vi "hamamatsu_dcam_update_camera_settings.vi"(6 "error in (no error)":errorcluster, 9 "Handle in":u32) -> (0 "error out":errorcluster, 3 "Handle out":u32)   [LabVIEW 2015]
panel:
  out "Display":T1(plugin-control)
  out "Software FPS":dbl
  out "Camera FPS":dbl
  out "SMD":dbl
  in  "Scan Mode":dbl min=1.0 max=2.0 step=1.0
  in  "Exposure":dbl min=0.0010036691729323308 max=10.000004210526315 step=1e-08
  out "EXP":dbl
  out "SVW":i32
  out "SHW":i32
  out "SVO":i32
  out "SHO":i32
  in  "V Width":i32 min=4 max=1124 step=4
  in  "V Offset":i32 min=0 max=1848 step=4
  in  "H Width":i32 min=4 max=2048 step=4
  in  "H Offset":i32 min=0 max=0 step=4
  in  "Binning":u16(ring)=1 items=["1x1"=1, "2x2"=2, "4x4"=4]
  out "Elapsed Time":u32
  out "Total Frames":i32
  in  "Display":bool=TRUE
  in  "continue":bool
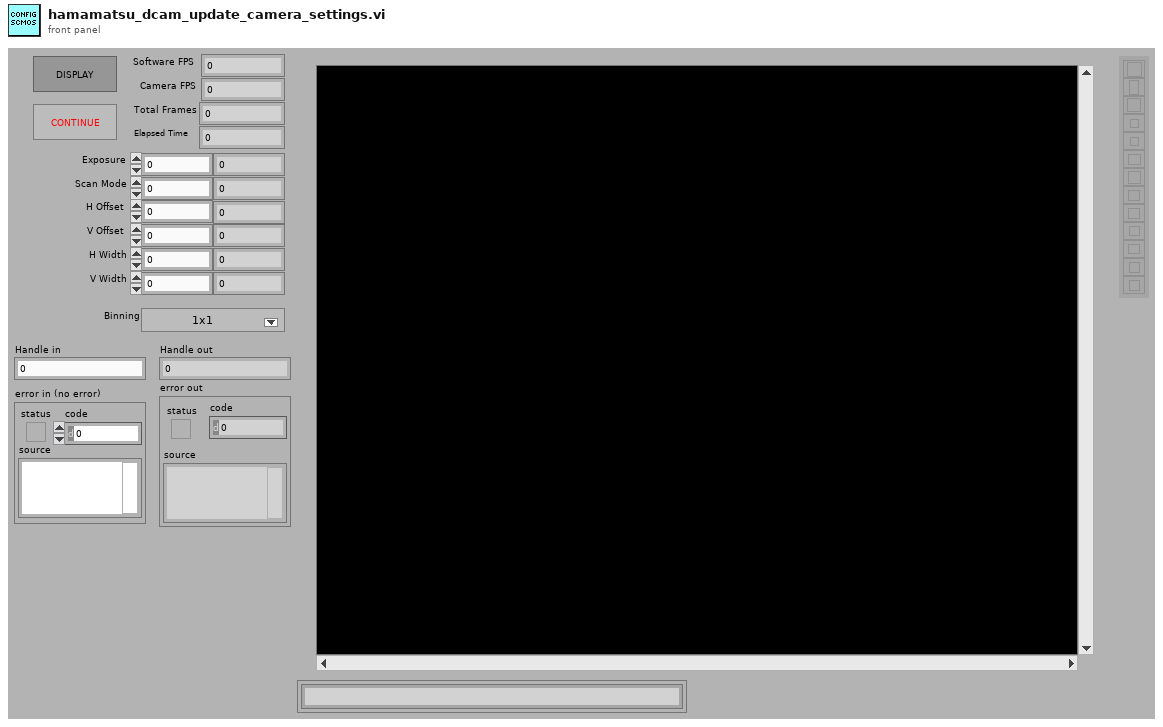
[diagram p1: front panel]
types:
  T1 = typedef "IMAQ Image.ctl" = refnum<image>
  T2 = typedef "Image Type" = u32
  T3 = cluster{"Value":i32, "Minimum":i32, "Maximum":i32, "Increment":i32}
  T4 = cluster{"height":u32, "width":u32, "datatype":u32}
  T5 = cluster{"H Offset":i32, "V Offset":i32, "H Width":i32, "V Width":i32}
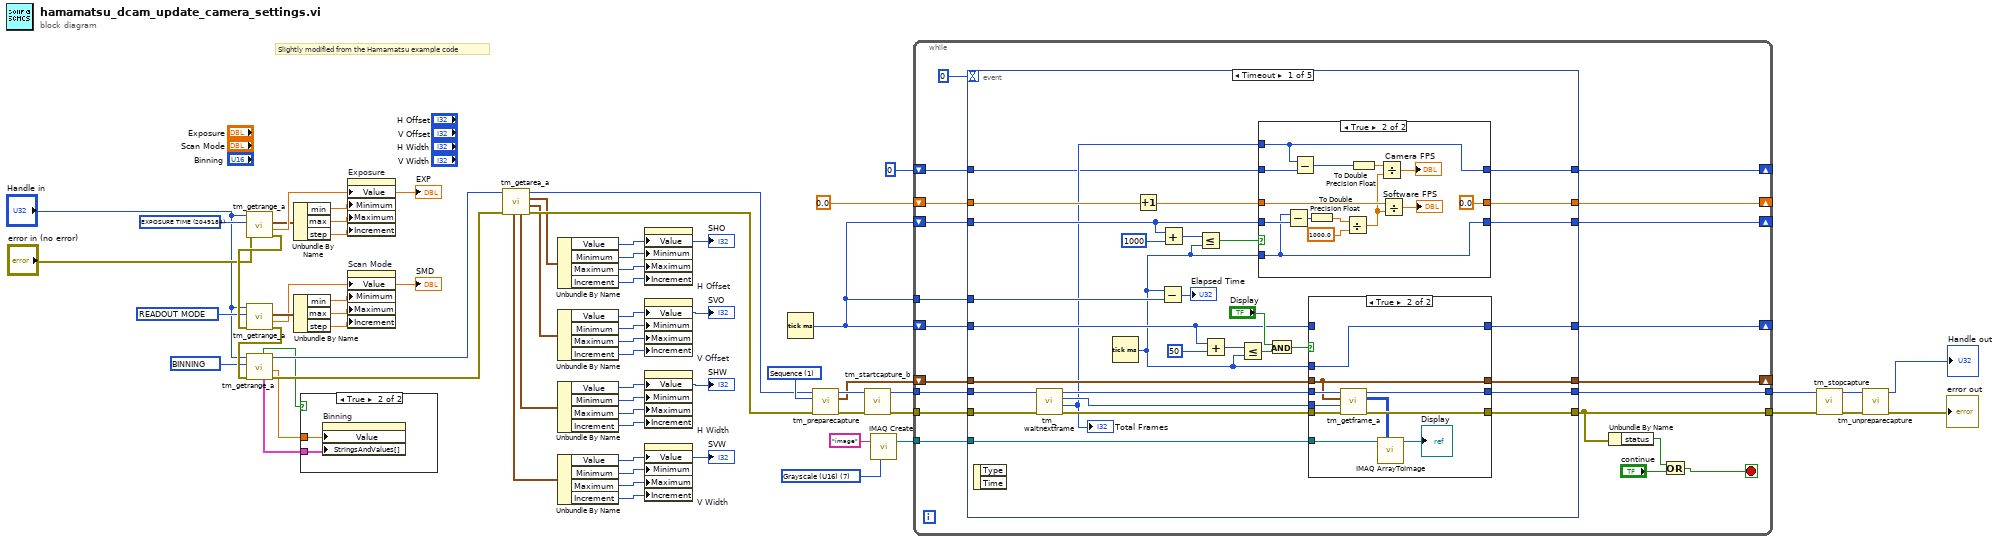
[diagram p0: block diagram]
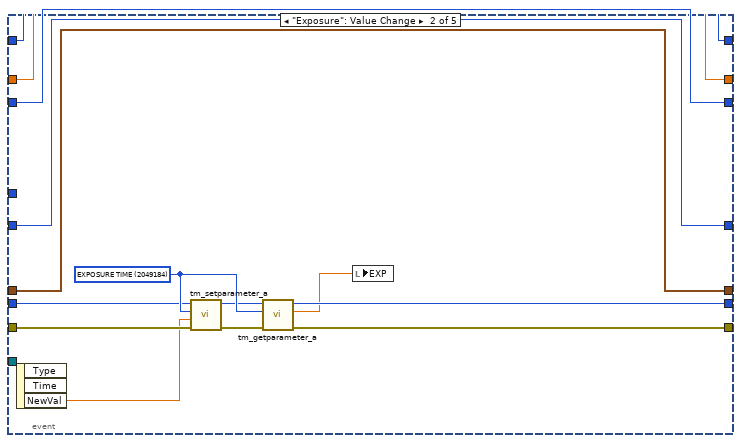
[diagram p5: hidden frame]
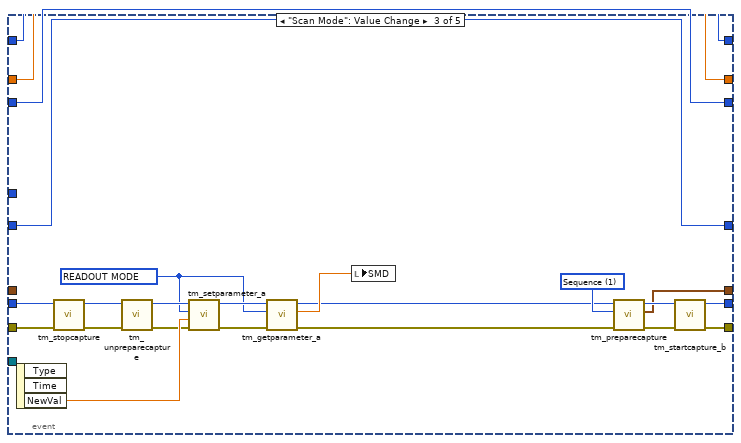
[diagram p6: hidden frame]
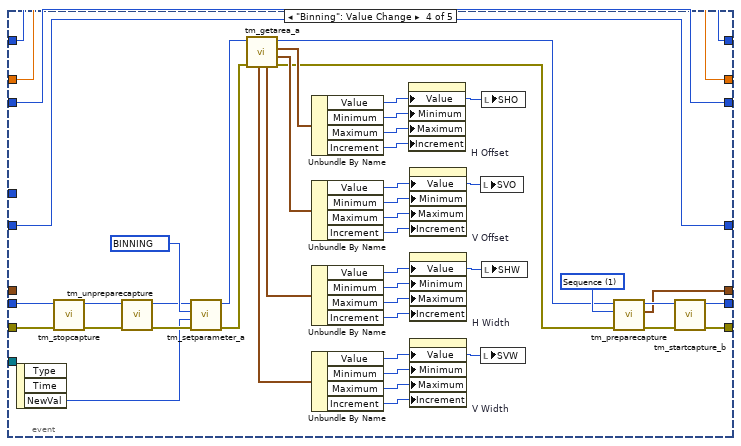
[diagram p7: hidden frame]
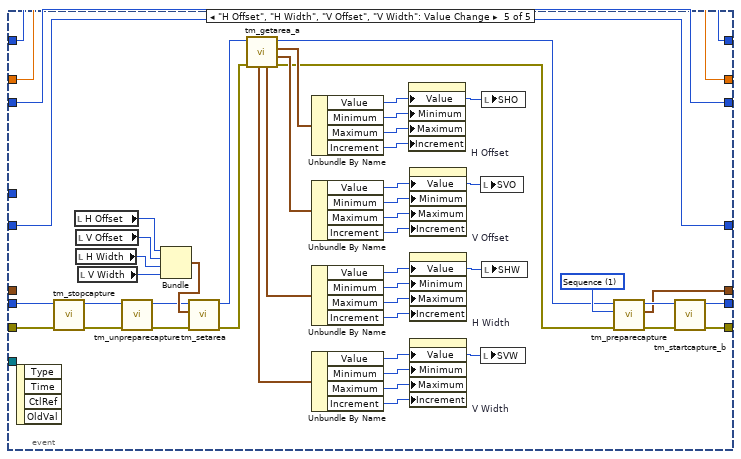
[diagram p8: hidden frame]
diagram:
  w8 = T2 7 items=["Grayscale (U8)", "Grayscale (I16)", "Grayscale (SGL)", "Complex (CSG)", "RGB (U32)", "HSL (U32)", "RGB (U64)", "Grayscale (U16)"] ("Image Type")
  w10 = u32 2049184 items=["BINNING"=4215968, "BITS PER CHANNEL"=4342976, "ACTIVE VIEW INDEX"=4343136, "CCD MODE"=4212384, "SENSOR MODE"=4212128, "READOUT MODE"=4211872, "EXPOSURE TIME"=2049184, "CONTRAST GAIN"=3163312, "CONTRAST OFFSET"=3163328, "LIGHT MODE"=2114720, "SENSITIVITY"=2114992, "WHITE BALANCE"=3163568, "PHOTON IMAGING MODE"=2115200, "HIGH DYNAMIC RANGE MODE"=3163360, "TRIGGER SOURCE"=1066144, "TRIGGER ACTIVE"=1066160, "TRIGGER MODE"=1066400, "TRIGGER POLARITY"=1066416, "TRIGGER GLOBAL EXPOSURE"=2049680, "FIRST TRIGGER BEHAVIOR"=2049696, "TRIGGER TIMES"=1066448, "OUTPUT TRIGGER POLARITY"=1852592, "OUTPUT TRIGGER DELAY"=1852624, "OUTPUT TRIGGER PERIOD"=1852640, "TEMPERATURE"=2115232, "TEMPERATURE TARGET"=2115264, "SENSOR COOLER FAN"=2115296, "MECHANICAL SHUTTER"=2115488, "BACK FOCUS POSITION"=8422304, "FRAMEBUNDLE MODE"=4346784, "FRAMEBUNDLE NUMBER"=4346800, "LINEBUNDLE HEIGHT"=4212192, "TRIGGER CONNECTOR"=1066432, "IMAGE PIXEL TYPE"=4343296, "OUTPUT TRIGGER KIND"=1852656, "READOUT DIRECTION"=4211904, "CHANNEL SYNC"=1852352] ("Parameter")
  w11 = u32 4211872 items=["BINNING"=4215968, "BITS PER CHANNEL"=4342976, "ACTIVE VIEW INDEX"=4343136, "CCD MODE"=4212384, "SENSOR MODE"=4212128, "READOUT MODE"=4211872, "EXPOSURE TIME"=2049184, "CONTRAST GAIN"=3163312, "CONTRAST OFFSET"=3163328, "LIGHT MODE"=2114720, "SENSITIVITY"=2114992, "WHITE BALANCE"=3163568, "PHOTON IMAGING MODE"=2115200, "HIGH DYNAMIC RANGE MODE"=3163360, "TRIGGER SOURCE"=1066144, "TRIGGER ACTIVE"=1066160, "TRIGGER MODE"=1066400, "TRIGGER POLARITY"=1066416, "TRIGGER GLOBAL EXPOSURE"=2049680, "FIRST TRIGGER BEHAVIOR"=2049696, "TRIGGER TIMES"=1066448, "OUTPUT TRIGGER POLARITY"=1852592, "OUTPUT TRIGGER DELAY"=1852624, "OUTPUT TRIGGER PERIOD"=1852640, "TEMPERATURE"=2115232, "TEMPERATURE TARGET"=2115264, "SENSOR COOLER FAN"=2115296, "MECHANICAL SHUTTER"=2115488, "BACK FOCUS POSITION"=8422304, "FRAMEBUNDLE MODE"=4346784, "FRAMEBUNDLE NUMBER"=4346800, "LINEBUNDLE HEIGHT"=4212192, "TRIGGER CONNECTOR"=1066432, "IMAGE PIXEL TYPE"=4343296, "OUTPUT TRIGGER KIND"=1852656, "READOUT DIRECTION"=4211904, "CHANNEL SYNC"=1852352] ("Parameter")
  w12 = u32 4215968 items=["BINNING"=4215968, "BITS PER CHANNEL"=4342976, "ACTIVE VIEW INDEX"=4343136, "CCD MODE"=4212384, "SENSOR MODE"=4212128, "READOUT MODE"=4211872, "EXPOSURE TIME"=2049184, "CONTRAST GAIN"=3163312, "CONTRAST OFFSET"=3163328, "LIGHT MODE"=2114720, "SENSITIVITY"=2114992, "WHITE BALANCE"=3163568, "PHOTON IMAGING MODE"=2115200, "HIGH DYNAMIC RANGE MODE"=3163360, "TRIGGER SOURCE"=1066144, "TRIGGER ACTIVE"=1066160, "TRIGGER MODE"=1066400, "TRIGGER POLARITY"=1066416, "TRIGGER GLOBAL EXPOSURE"=2049680, "FIRST TRIGGER BEHAVIOR"=2049696, "TRIGGER TIMES"=1066448, "OUTPUT TRIGGER POLARITY"=1852592, "OUTPUT TRIGGER DELAY"=1852624, "OUTPUT TRIGGER PERIOD"=1852640, "TEMPERATURE"=2115232, "TEMPERATURE TARGET"=2115264, "SENSOR COOLER FAN"=2115296, "MECHANICAL SHUTTER"=2115488, "BACK FOCUS POSITION"=8422304, "FRAMEBUNDLE MODE"=4346784, "FRAMEBUNDLE NUMBER"=4346800, "LINEBUNDLE HEIGHT"=4212192, "TRIGGER CONNECTOR"=1066432, "IMAGE PIXEL TYPE"=4343296, "OUTPUT TRIGGER KIND"=1852656, "READOUT DIRECTION"=4211904, "CHANNEL SYNC"=1852352] ("Parameter")
  w61 = 1 items=["Snap", "Sequence"] ("Capture mode")
  # "Slightly modified from the Hamamatsu example code"
  n1 = call <userlib>:"tm_getrange_a.vi"("error in (no error)"="error in (no error)", "Parameter"=w10, "Handle in"="Handle in") -> ("error out"=w21:errorcluster, "default"=w23:dbl, "Range"=w22:cluster{"min":dbl, "max":dbl, "step":dbl})  [unwired: 2 in, 4 out]
  "EXP" <- w23
  n2 = call <userlib>:"tm_getrange_a.vi"("error in (no error)"=w21, "Parameter"=w11, "Handle in"="Handle in") -> ("error out"=w18:errorcluster, "default"=w19:dbl, "Range"=w20:cluster{"min":dbl, "max":dbl, "step":dbl})  [unwired: 2 in, 4 out]
  "SMD" <- w19
  n3 = call <userlib>:"tm_getrange_a.vi"("error in (no error)"=w18, "Parameter"=w12, "Handle in"="Handle in") -> ("error out"=w17:errorcluster, "default"=w14:dbl, "Handle out"=w16:u32, "Value Names"=w13:cluster{"Name":string, "Value":dbl}[], "Writable"=w15:bool)  [unwired: 2 in, 2 out]
  n4 = Unbundle By Name(w22) -> ("min"=w54:dbl, "max"=w53:dbl, "step"=w52:dbl)
  n5 = Unbundle By Name(w20) -> ("min"=w51:dbl, "max"=w50:dbl, "step"=w49:dbl)
  n6 = case shown="True" w15 {
    tunnel: w13 -> [_ w64]
    tunnel: w14 -> [_ w63]
    frame False {
    }
    frame True {
      n7 = property on="Binning" class="Ring (strict)"("Value"=w63, "StringsAndValues[]"=w64) -> ()  [unwired: 2 in, 2 out]
    }
  }
  n8 = property on="Exposure" class="DigNum (strict)"("Value"=w23, "Minimum"=w54, "Maximum"=w53, "Increment"=w52) -> ()  [unwired: 2 in, 2 out]
  n9 = property on="Scan Mode" class="DigNum (strict)"("Value"=w19, "Minimum"=w51, "Maximum"=w50, "Increment"=w49) -> ()  [unwired: 2 in, 2 out]
  n10 = call <userlib>:"tm_getarea_a.vi"("error in (no error)"=w17, "Handle in"=w16) -> ("error out"=w47:errorcluster, "V Offset"=w46:T3, "H Offset"=w29:T3, "Handle out"=w48:u32, "H Width"=w45:T3, "V Width"=w44:T3)  [unwired: 4 in]
  n11 = Unbundle By Name(w29) -> ("Value"=w28:i32, "Minimum"=w27:i32, "Maximum"=w26:i32, "Increment"=w25:i32)
  "SHO" <- w28
  n12 = Unbundle By Name(w46) -> ("Value"=w34:i32, "Minimum"=w43:i32, "Maximum"=w42:i32, "Increment"=w41:i32)
  "SVO" <- w34
  n13 = Unbundle By Name(w45) -> ("Value"=w33:i32, "Minimum"=w40:i32, "Maximum"=w39:i32, "Increment"=w38:i32)
  "SHW" <- w33
  n14 = Unbundle By Name(w44) -> ("Value"=w32:i32, "Minimum"=w37:i32, "Maximum"=w36:i32, "Increment"=w35:i32)
  "SVW" <- w32
  n15 = property on="H Offset" class="DigNum (strict)"("Value"=w28, "Minimum"=w27, "Maximum"=w26, "Increment"=w25) -> ()  [unwired: 2 in, 2 out]
  n16 = property on="V Offset" class="DigNum (strict)"("Value"=w34, "Minimum"=w43, "Maximum"=w42, "Increment"=w41) -> ()  [unwired: 2 in, 2 out]
  n17 = property on="H Width" class="DigNum (strict)"("Value"=w33, "Minimum"=w40, "Maximum"=w39, "Increment"=w38) -> ()  [unwired: 2 in, 2 out]
  n18 = property on="V Width" class="DigNum (strict)"("Value"=w32, "Minimum"=w37, "Maximum"=w36, "Increment"=w35) -> ()  [unwired: 2 in, 2 out]
  n19 = Tick Count (ms)() -> (millisecond timer value=w55:u32)
  n20 = call <userlib>:"tm_preparecapture.vi"("error in (no error)"=w47, "Capture mode"=w61, "Handle in"=w48) -> ("error out"=w59:errorcluster, "Buffer Info"=w56:T4, "Handle out"=w60:u32)  [unwired: 5 in, 1 out]
  n21 = call <userlib>:"tm_startcapture_b.vi"("error in (no error)"=w59, "Handle in"=w60) -> ("error out"=w58:errorcluster, "Handle out"=w57:u32)  [unwired: 8 in]
  n22 = call "IMAQ Create"("Image Name"="image", "Image Type"=w8) -> ("New Image"=w7:T1)  [unwired: 3 in, 1 out]
  n23 = while {
    tunnel: w58 -> [w74]
    tunnel: [w72] -> w31
    tunnel: [w71] -> w30
    shift-right: [w81] -> _
    shift-left: w55 -> [w79]
    shift-right: [w82] -> _
    shift-left: 0.0 -> [w80]
    shift-right: [w73] -> _
    shift-left: w55 -> [w77]
    tunnel: w57 -> [w75]
    tunnel: w55 -> [w78]
    shift-right: [w70] -> _
    shift-left: w56 -> [w76]
    shift-right: [w67] -> _
    shift-left: 0 -> [w68]
    tunnel: w7 -> [w66]
    stop <- w65 stop-if-true
    n24 = event shown="[0] Timeout" {
      selector: _ -> [_ _ _ _ _]
      dyn-events: _ -> [_ _ _ _ _]
      timeout: 0 -> [_ _ _ _ _]
      tunnel: [w90 w158 w181 w217 w262] -> w82
      tunnel: [w89 w159 w182 w218 w263] -> w81
      tunnel: w80 -> [w101 w158 w181 w217 w262]
      tunnel: w79 -> [w92 w159 w182 w218 w263]
      tunnel: w78 -> [w97 _ _ _ _]
      tunnel: w77 -> [w102 w160 w183 w225 w270]
      tunnel: w76 -> [w96 w157 _ _ _]
      tunnel: w75 -> [w104 w152 w178 w194 w232]
      tunnel: w74 -> [w103 w154 w177 w193 w231]
      tunnel: [w100 w160 w183 w225 w270] -> w73
      tunnel: [w99 w149 w172 w220 w265] -> w72
      tunnel: [w98 w147 w173 w221 w266] -> w71
      tunnel: [w95 w157 w171 w219 w264] -> w70
      tunnel: w68 -> [w87 w156 w170 w190 w226]
      tunnel: [w86 w156 w170 w190 w226] -> w67
      tunnel: w66 -> [w85 _ _ _ _]
      event Timeout {
        n25 = event-data() -> ()  [unwired: 1 in, 2 out]
        n26 = call <userlib>:"tm_waitnextframe.vi"("error in (no error)"=w103, "Handle in"=w104) -> ("error out"=w108:errorcluster, "Frame Count"=w88:i32, "Frame Index"=w107:i32, "Handle out"=w109:u32)  [unwired: 6 in]
        "Total Frames" <- w88
        n27 = Tick Count (ms)() -> (millisecond timer value=w94:u32)
        n28 = Increment(x=w101) -> (x+1=w91:dbl)
        n29 = Subtract(x=w94, y=w97) -> (x-y=→"Elapsed Time":u32)
        n30 = Add(x=w92, y=u32 1000) -> (x+y=w115:u32)
        n31 = Less Or Equal?(x=w115, y=w94) -> (x <= y?=w93:bool)
        n32 = Add(x=w102, y=u32 50) -> (x+y=w113:u32)
        n33 = Less Or Equal?(x=w113, y=w94) -> (x <= y?=w111:bool)
        n34 = case shown="True" w93 {
          tunnel: w92 -> [w118 w127]
          tunnel: [w118 w124] -> w89
          tunnel: w91 -> [w117 w130]
          tunnel: w94 -> [_ w124]
          tunnel: [w117 0.0] -> w90
          tunnel: w88 -> [_ w119]
          tunnel: w87 -> [w116 w122]
          tunnel: [w116 w119] -> w86
          frame False {
          }
          frame True {
            n35 = Subtract(x=w124, y=w127) -> (x-y=w126:u32)
            n36 = Subtract(x=w119, y=w122) -> (x-y=w120:i32)
            n37 = To Double Precision Float(number=w126) -> (double precision float=w132:dbl)
            n38 = Divide(x=w132, y=1000.0) -> (x/y=w123:dbl)
            n39 = To Double Precision Float(number=w120) -> (double precision float=w121:dbl)
            n40 = Divide(x=w121, y=w123) -> (x/y=→"Camera FPS":dbl)
            n41 = Divide(x=w130, y=w123) -> (x/y=→"Software FPS":dbl)
          }
        }
        n42 = And(x="Display", y=w111) -> (x .and. y?=w106:bool)
        n43 = case shown="True" w106 {
          tunnel: w102 -> [w136 _]
          tunnel: w94 -> [_ w146]
          tunnel: [w136 w146] -> w100
          tunnel: w109 -> [w135 w145]
          tunnel: w96 -> [w133 w140]
          tunnel: w108 -> [w134 w144]
          tunnel: [w135 w143] -> w99
          tunnel: [w134 w142] -> w98
          tunnel: w107 -> [_ w141]
          tunnel: [w133 w140] -> w95
          tunnel: w85 -> [_ w138]
          frame False {
          }
          frame True {
            n44 = call <userlib>:"tm_getframe_a.vi"("error in (no error)"=w144, "Frame Index"=w141, "Buffer Info"=w140, "Handle in"=w145) -> ("error out"=w142:errorcluster, "Data 16"=w139:u16[][], "Handle out"=w143:u32)  [unwired: 3 in, 2 out]
            n45 = call "IMAQ ArrayToImage"("Image Pixels (U16)"=w139, "Image"=w138) -> ("Image Out"=→"Display":T1)  [unwired: 8 in, 1 out]
          }
        }
      }
      event "Exposure": Value Change {
        w155 = u32 2049184 items=["SENSOR MODE"=4212128, "CCD MODE"=4212384, "READOUT MODE"=4211872, "ACTIVE VIEW INDEX"=4343136, "BITS PER CHANNEL"=4342976, "IMAGE PIXEL TYPE"=4343296, "BINNING"=4215968, "EXPOSURE TIME"=2049184, "CONTRAST GAIN"=3163312, "CONTRAST OFFSET"=3163328, "LIGHT MODE"=2114720, "SENSITIVITY"=2114992, "PHOTON IMAGING MODE"=2115200, "HIGH DYNAMIC RANGE MODE"=3163360, "WHITE BALANCE"=3163568, "TEMPERATURE"=2115232, "TEMPERATURE TARGET"=2115264, "SENSOR COOLER FAN"=2115296, "LINEBUNDLE HEIGHT"=4212192, "MECHANICAL SHUTTER"=2115488, "BACK FOCUS POSITION"=8422304, "TRIGGER CONNECTOR"=1066432, "TRIGGER SOURCE"=1066144, "OUTPUT TRIGGER SOURCE"=1852576, "TRIGGER GLOBAL EXPOSURE"=2049680, "FIRST TRIGGER BEHAVIOR"=2049696, "CHANNEL SYNC"=1852352, "READOUT DIRECTION"=4211904, "PRE HSYNC COUNT"=1852704] ("Parameter")
        n46 = event-data() -> ("NewVal"=w153:dbl)  [unwired: 1 in, 2 out]
        n47 = call <userlib>:"tm_setparameter_a.vi"("error in (no error)"=w154, "Value in"=w153, "Parameter"=w155, "Handle in"=w152) -> ("error out"=w151:errorcluster, "Handle out"=w150:u32)  [unwired: 6 in]
        n48 = call <userlib>:"tm_getparameter_a.vi"("error in (no error)"=w151, "Parameter"=w155, "Handle in"=w150) -> ("error out"=w147:errorcluster, "Value out"=w148:dbl, "Handle out"=w149:u32)  [unwired: 6 in]
        n49 = local write "EXP"(w148) -> ()
      }
      event "Scan Mode": Value Change {
        w161 = u32 4211872 items=["SENSOR MODE"=4212128, "CCD MODE"=4212384, "READOUT MODE"=4211872, "ACTIVE VIEW INDEX"=4343136, "BITS PER CHANNEL"=4342976, "IMAGE PIXEL TYPE"=4343296, "BINNING"=4215968, "EXPOSURE TIME"=2049184, "CONTRAST GAIN"=3163312, "CONTRAST OFFSET"=3163328, "LIGHT MODE"=2114720, "SENSITIVITY"=2114992, "PHOTON IMAGING MODE"=2115200, "HIGH DYNAMIC RANGE MODE"=3163360, "WHITE BALANCE"=3163568, "TEMPERATURE"=2115232, "TEMPERATURE TARGET"=2115264, "SENSOR COOLER FAN"=2115296, "LINEBUNDLE HEIGHT"=4212192, "MECHANICAL SHUTTER"=2115488, "BACK FOCUS POSITION"=8422304, "TRIGGER CONNECTOR"=1066432, "TRIGGER SOURCE"=1066144, "OUTPUT TRIGGER SOURCE"=1852576, "TRIGGER GLOBAL EXPOSURE"=2049680, "FIRST TRIGGER BEHAVIOR"=2049696, "CHANNEL SYNC"=1852352, "READOUT DIRECTION"=4211904, "PRE HSYNC COUNT"=1852704] ("Parameter")
        w176 = 1 items=["Snap", "Sequence"] ("Capture mode")
        n50 = event-data() -> ("NewVal"=w166:dbl)  [unwired: 1 in, 2 out]
        n51 = call <userlib>:"tm_stopcapture.vi"("error in (no error)"=w177, "Handle in"=w178) -> ("error out"=w179:errorcluster, "Handle out"=w180:u32)  [unwired: 8 in]
        n52 = call <userlib>:"tm_unpreparecapture.vi"("error in (no error)"=w179, "Handle in"=w180) -> ("error out"=w164:errorcluster, "Handle out"=w165:u32)  [unwired: 8 in]
        n53 = call <userlib>:"tm_setparameter_a.vi"("error in (no error)"=w164, "Value in"=w166, "Parameter"=w161, "Handle in"=w165) -> ("error out"=w163:errorcluster, "Handle out"=w162:u32)  [unwired: 6 in]
        n54 = call <userlib>:"tm_getparameter_a.vi"("error in (no error)"=w163, "Parameter"=w161, "Handle in"=w162) -> ("error out"=w169:errorcluster, "Value out"=w168:dbl, "Handle out"=w167:u32)  [unwired: 6 in]
        n55 = local write "SMD"(w168) -> ()
        n56 = call <userlib>:"tm_preparecapture.vi"("error in (no error)"=w169, "Capture mode"=w176, "Handle in"=w167) -> ("error out"=w174:errorcluster, "Buffer Info"=w171:T4, "Handle out"=w175:u32)  [unwired: 5 in, 1 out]
        n57 = call <userlib>:"tm_startcapture_b.vi"("error in (no error)"=w174, "Handle in"=w175) -> ("error out"=w173:errorcluster, "Handle out"=w172:u32)  [unwired: 8 in]
      }
      event "Binning": Value Change {
        w185 = u32 4215968 items=["BINNING"=4215968, "BITS PER CHANNEL"=2, "ACTIVE VIEW INDEX"=3, "CCD MODE"=4, "SENSOR MODE"=5, "READOUT MODE"=6, "EXPOSURE TIME"=7, "CONTRAST GAIN"=8, "CONTRAST OFFSET"=9, "LIGHT MODE"=10, "SENSITIVITY"=11, "WHITE BALANCE"=12, "PHOTON IMAGING MODE"=13, "HIGH DYNAMIC RANGE MODE"=14, "TRIGGER SOURCE"=15, "TRIGGER ACTIVE"=16, "TRIGGER MODE"=17, "TRIGGER POLARITY"=18, "TRIGGER GLOBAL EXPOSURE"=19, "FIRST TRIGGER BEHAVIOR"=20, "TRIGGER TIMES"=21, "OUTPUT TRIGGER POLARITY"=22, "OUTPUT TRIGGER DELAY"=23, "OUTPUT TRIGGER PERIOD"=24, "TEMPERATURE"=25, "TEMPERATURE TARGET"=26, "SENSOR COOLER FAN"=27, "MECHANICAL SHUTTER"=28, "BACK FOCUS POSITION"=29, "FRAMEBUNDLE MODE"=30, "FRAMEBUNDLE NUMBER"=31, "LINEBUNDLE HEIGHT"=32, "TRIGGER CONNECTOR"=33, "IMAGE PIXEL TYPE"=34, "OUTPUT TRIGGER KIND"=35, "READOUT DIRECTION"=36, "CHANNEL SYNC"=37] ("Parameter")
        w224 = 1 items=["Snap", "Sequence"] ("Capture mode")
        n58 = event-data() -> ("NewVal"=w186:u16)  [unwired: 1 in, 2 out]
        n59 = call <userlib>:"tm_stopcapture.vi"("error in (no error)"=w193, "Handle in"=w194) -> ("error out"=w191:errorcluster, "Handle out"=w192:u32)  [unwired: 8 in]
        n60 = call <userlib>:"tm_unpreparecapture.vi"("error in (no error)"=w191, "Handle in"=w192) -> ("error out"=w187:errorcluster, "Handle out"=w184:u32)  [unwired: 8 in]
        n61 = call <userlib>:"tm_setparameter_a.vi"("error in (no error)"=w187, "Value in"=w186, "Parameter"=w185, "Handle in"=w184) -> ("error out"=w188:errorcluster, "Handle out"=w189:u32)  [unwired: 6 in]
        n62 = call <userlib>:"tm_getarea_a.vi"("error in (no error)"=w188, "Handle in"=w189) -> ("error out"=w212:errorcluster, "V Offset"=w214:T3, "H Offset"=w213:T3, "Handle out"=w211:u32, "H Width"=w215:T3, "V Width"=w216:T3)  [unwired: 4 in]
        n63 = Unbundle By Name(w213) -> ("Value"=w207:i32, "Minimum"=w210:i32, "Maximum"=w209:i32, "Increment"=w208:i32)
        n64 = Unbundle By Name(w214) -> ("Value"=w197:i32, "Minimum"=w206:i32, "Maximum"=w205:i32, "Increment"=w204:i32)
        n65 = Unbundle By Name(w215) -> ("Value"=w196:i32, "Minimum"=w203:i32, "Maximum"=w202:i32, "Increment"=w201:i32)
        n66 = Unbundle By Name(w216) -> ("Value"=w195:i32, "Minimum"=w200:i32, "Maximum"=w199:i32, "Increment"=w198:i32)
        n67 = property on="H Offset" class="DigNum (strict)"("Value"=w207, "Minimum"=w210, "Maximum"=w209, "Increment"=w208) -> ()  [unwired: 2 in, 2 out]
        n68 = property on="V Offset" class="DigNum (strict)"("Value"=w197, "Minimum"=w206, "Maximum"=w205, "Increment"=w204) -> ()  [unwired: 2 in, 2 out]
        n69 = property on="H Width" class="DigNum (strict)"("Value"=w196, "Minimum"=w203, "Maximum"=w202, "Increment"=w201) -> ()  [unwired: 2 in, 2 out]
        n70 = property on="V Width" class="DigNum (strict)"("Value"=w195, "Minimum"=w200, "Maximum"=w199, "Increment"=w198) -> ()  [unwired: 2 in, 2 out]
        n71 = local write "SVO"(w197) -> ()
        n72 = local write "SVW"(w195) -> ()
        n73 = local write "SHO"(w207) -> ()
        n74 = local write "SHW"(w196) -> ()
        n75 = call <userlib>:"tm_preparecapture.vi"("error in (no error)"=w212, "Capture mode"=w224, "Handle in"=w211) -> ("error out"=w222:errorcluster, "Buffer Info"=w219:T4, "Handle out"=w223:u32)  [unwired: 5 in, 1 out]
        n76 = call <userlib>:"tm_startcapture_b.vi"("error in (no error)"=w222, "Handle in"=w223) -> ("error out"=w221:errorcluster, "Handle out"=w220:u32)  [unwired: 8 in]
      }
      event "H Offset", "H Width", "V Offset", "V Width": Value Change {
        w269 = 1 items=["Snap", "Sequence"] ("Capture mode")
        n77 = event-data() -> ()  [unwired: 1 in, 4 out]
        n78 = call <userlib>:"tm_stopcapture.vi"("error in (no error)"=w231, "Handle in"=w232) -> ("error out"=w229:errorcluster, "Handle out"=w230:u32)  [unwired: 8 in]
        n79 = local read "H Offset"() -> (w235:i32)
        n80 = local read "V Offset"() -> (w237:i32)
        n81 = local read "H Width"() -> (w236:i32)
        n82 = local read "V Width"() -> (w234:i32)
        n83 = call <userlib>:"tm_unpreparecapture.vi"("error in (no error)"=w229, "Handle in"=w230) -> ("error out"=w227:errorcluster, "Handle out"=w228:u32)  [unwired: 8 in]
        n84 = Bundle("H Offset"=w235, "V Offset"=w237, "H Width"=w236, "V Width"=w234) -> (w233:T5)  [unwired: 1 in]
        n85 = call <userlib>:"tm_setarea.vi"("error in (no error)"=w227, "Sub Region"=w233, "Handle in"=w228) -> ("error out"=w238:errorcluster, "Handle out"=w239:u32)  [unwired: 7 in]
        n86 = call <userlib>:"tm_getarea_a.vi"("error in (no error)"=w238, "Handle in"=w239) -> ("error out"=w257:errorcluster, "V Offset"=w259:T3, "H Offset"=w258:T3, "Handle out"=w256:u32, "H Width"=w260:T3, "V Width"=w261:T3)  [unwired: 4 in]
        n87 = Unbundle By Name(w258) -> ("Value"=w252:i32, "Minimum"=w255:i32, "Maximum"=w254:i32, "Increment"=w253:i32)
        n88 = Unbundle By Name(w259) -> ("Value"=w242:i32, "Minimum"=w251:i32, "Maximum"=w250:i32, "Increment"=w249:i32)
        n89 = Unbundle By Name(w260) -> ("Value"=w241:i32, "Minimum"=w248:i32, "Maximum"=w247:i32, "Increment"=w246:i32)
        n90 = Unbundle By Name(w261) -> ("Value"=w240:i32, "Minimum"=w245:i32, "Maximum"=w244:i32, "Increment"=w243:i32)
        n91 = property on="H Offset" class="DigNum (strict)"("Value"=w252, "Minimum"=w255, "Maximum"=w254, "Increment"=w253) -> ()  [unwired: 2 in, 2 out]
        n92 = property on="V Offset" class="DigNum (strict)"("Value"=w242, "Minimum"=w251, "Maximum"=w250, "Increment"=w249) -> ()  [unwired: 2 in, 2 out]
        n93 = property on="H Width" class="DigNum (strict)"("Value"=w241, "Minimum"=w248, "Maximum"=w247, "Increment"=w246) -> ()  [unwired: 2 in, 2 out]
        n94 = property on="V Width" class="DigNum (strict)"("Value"=w240, "Minimum"=w245, "Maximum"=w244, "Increment"=w243) -> ()  [unwired: 2 in, 2 out]
        n95 = local write "SVO"(w242) -> ()
        n96 = local write "SVW"(w240) -> ()
        n97 = local write "SHO"(w252) -> ()
        n98 = local write "SHW"(w241) -> ()
        n99 = call <userlib>:"tm_preparecapture.vi"("error in (no error)"=w257, "Capture mode"=w269, "Handle in"=w256) -> ("error out"=w267:errorcluster, "Buffer Info"=w264:T4, "Handle out"=w268:u32)  [unwired: 5 in, 1 out]
        n100 = call <userlib>:"tm_startcapture_b.vi"("error in (no error)"=w267, "Handle in"=w268) -> ("error out"=w266:errorcluster, "Handle out"=w265:u32)  [unwired: 8 in]
      }
    }
    n101 = Unbundle By Name(w71) -> ("status"=w83:bool)
    n102 = Or(x=w83, y="continue") -> (x .or. y?=w65:bool)
  }
  n103 = call <userlib>:"tm_stopcapture.vi"("error in (no error)"=w30, "Handle in"=w31) -> ("error out"=w4:errorcluster, "Handle out"=w3:u32)  [unwired: 8 in]
  n104 = call <userlib>:"tm_unpreparecapture.vi"("error in (no error)"=w4, "Handle in"=w3) -> ("error out"=→"error out":errorcluster, "Handle out"=→"Handle out":u32)  [unwired: 8 in]
